vi "Read Current Laser Power.vi"(8 "error in (no error)":errorcluster, 11 "Test Station SIM Laser Driver in":refnum<class "Test Station SIM Laser Driver.lvclass">) -> (0 "error out":errorcluster, 2 "Current Laser Power":dbl, 3 "Test Station SIM Laser Driver out":refnum<class "Test Station SIM Laser Driver.lvclass">)   [LabVIEW 2022 SP3, in "Test Station SIM Laser Driver.lvclass"]
uses:
  Test Station SIM Laser Driver.lvclass
  Action.ctl
  Sim Laser Driver/Sim Laser Driver.lvclass
  Test Station SIM Laser Driver.lvclass/Test Station SIM Laser Driver.ctl
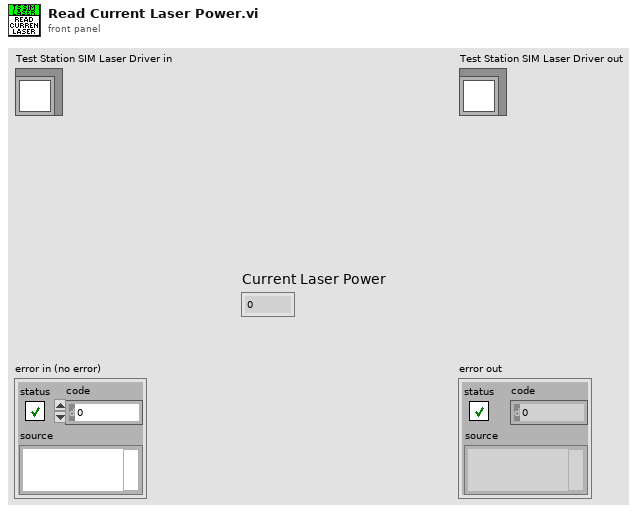
[diagram p1: front panel]
types:
  T1 = typedef "Test Station SIM Laser Driver.lvclass/Action.ctl" = enum16{"Read Data", "Set Data"}
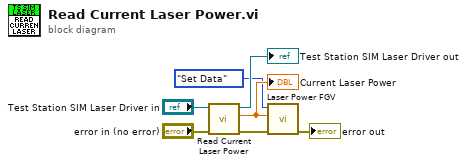
[diagram p0: block diagram]
diagram:
  n1 = call-parent "Read Current Laser Power.vi"("error in (no error)"="error in (no error)", "Sim Laser Driver in"="Test Station SIM Laser Driver in") -> ("error out"=w2:errorcluster, "Current Laser Power"=w4:dbl, "Sim Laser Driver out"=→"Test Station SIM Laser Driver out":refnum<class "Test Station SIM Laser Driver.lvclass">)  [unwired: 7 in]
  "Current Laser Power" <- w4
  n2 = call "Laser Power FGV.vi"("error in (no error)"=w2, "Laser Power"=w4, "Action"=Action."Set Data") -> ("error out"=→"error out":errorcluster)  [unwired: 7 in, 1 out]
